vi "play-with-variants_write_to_file.vi"() -> ()   [LabVIEW 2019]
uses:
  <vilib>/Utility/Data Type/Type Definitions/Data Type.ctl
  <vilib>/Utility/Data Type/Type Definitions/Type Definition Info.ctl
  <vilib>/Rock Robotics/SystemInterfaces/NetworkCommunication/NetComm_UsageReport_report.vi
  <vilib>/Rock Robotics/WPI/ThirdParty/JAS_Junk/TrajLib/DiffDriveKinematicsConstraint_New.vi
  <vilib>/Rock Robotics/WPI/ThirdParty/JAS_Junk/TrajLib/TrajectoryConfig_AddConstraint.vi
  <vilib>/Rock Robotics/WPI/ThirdParty/JAS_Junk/TrajLib/CentripetalAccelConstraint_New.vi
  <vilib>/Rock Robotics/WPI/ThirdParty/JAS_Junk/TrajLib/DiffDriveVoltageConstraint_New.vi
  <vilib>/Rock Robotics/WPI/ThirdParty/JAS_Junk/TrajLib/MecaDriveKinematicsConstraint_New.vi
  <vilib>/Rock Robotics/WPI/ThirdParty/JAS_Junk/TrajLib/SwerveDriveKinematicsConstraint_New.vi
  <vilib>/Rock Robotics/WPI/ThirdParty/JAS_Junk/TrajLib/Util_LibraryGlobals.vi
  <vilib>/Rock Robotics/WPI/ThirdParty/JAS_Junk/TrajLib/Trajectory_Library.lvlib
  <vilib>/Utility/Data Type/NI_Data Type.lvlib
  <vilib>/Rock Robotics/WPI/ThirdParty/JAS_Junk/TrajLib/TRAJ_CONSTRAINT_CENTRIPETAL_ACCEL.ctl
  <vilib>/Rock Robotics/WPI/ThirdParty/JAS_Junk/TrajLib/DIFF_DRIVE_KINEMATICS.ctl
  <vilib>/Rock Robotics/WPI/ThirdParty/JAS_Junk/TrajLib/TRAJ_CONSTRAINT_DIIF_DRIVE_KINEMATICS.ctl
  <vilib>/Rock Robotics/WPI/ThirdParty/JAS_Junk/TrajLib/TRANSLATION2D.ctl
  <vilib>/Analysis/Matrix/Datatypes/RealMatrix.ctl
  <vilib>/Analysis/Matrix/NI_Matrix.lvlib
  <vilib>/Rock Robotics/WPI/ThirdParty/JAS_Junk/TrajLib/MECA_DRIVE_KINEMATICS.ctl
  <vilib>/Rock Robotics/WPI/ThirdParty/JAS_Junk/TrajLib/TRAJ_CONSTRAINT_MECA_DRIVE_KINEMATICS.ctl
  <vilib>/Rock Robotics/WPI/ThirdParty/JAS_Junk/TrajLib/SWERVE_DRIVE_KINEMATICS.ctl
  <vilib>/Rock Robotics/WPI/ThirdParty/JAS_Junk/TrajLib/TRAJ_CONSTRAINT_SWERVE_DRIVE_KINEMATICS.ctl
  <vilib>/Rock Robotics/WPI/ThirdParty/JAS_Junk/TrajLib/SIMPLE_MOTOR_FF.ctl
  <vilib>/Rock Robotics/WPI/ThirdParty/JAS_Junk/TrajLib/TRAJ_CONSTRAINT_DIIF_DRIVE_VOLTAGE.ctl
  TrajConfig_XML_V5.ctl
panel:
  out "output cluster":T1 {"CentAccelConstraint"."Max Cent Accel" format="%20.4f"; "DiffDriveKineConstraint"."Max Accel (M/S2)" format="%20.4f"; "DiffDriveKineConstraint"."DIFF_DRIVE_KINEMATICS"."TrackWidth_Meters" format="%20.4f"; "DiffDriveKineConstraint"."Max Speed (M/S)" format="%20.4f"; "MecaKineConstraint"."MECA_DRIVE_KINEMATICS"."PrevCoR"."Y" format="%14.3f"; "MecaKineConstraint"."MECA_DRIVE_KINEMATICS"."PrevCoR"."X" format="%14.3f"; "MecaKineConstraint"."MECA_DRIVE_KINEMATICS"."RearRight"."Y" format="%14.3f"; "MecaKineConstraint"."MECA_DRIVE_KINEMATICS"."RearRight"."X" format="%14.3f"; "MecaKineConstraint"."MECA_DRIVE_KINEMATICS"."RearLeft"."Y" format="%14.3f"; "MecaKineConstraint"."MECA_DRIVE_KINEMATICS"."RearLeft"."X" format="%14.3f"; "MecaKineConstraint"."MECA_DRIVE_KINEMATICS"."FrontRight"."Y" format="%14.3f"; "MecaKineConstraint"."MECA_DRIVE_KINEMATICS"."FrontRight"."X" format="%14.3f"; "MecaKineConstraint"."MECA_DRIVE_KINEMATICS"."FrontLeft"."Y" format="%14.3f"; "MecaKineConstraint"."MECA_DRIVE_KINEMATICS"."FrontLeft"."X" format="%14.3f"; "MecaKineConstraint"."Max Speed (M/S)" format="%20.4f"; "SwerveKineConstraint"."SwerveKinematics"."PrevCoR"."Y" format="%14.3f"; "SwerveKineConstraint"."SwerveKinematics"."PrevCoR"."X" format="%14.3f"; "SwerveKineConstraint"."SwerveKinematics"."Modules"."Y" format="%14.3f"; "SwerveKineConstraint"."SwerveKinematics"."Modules"."X" format="%14.3f"; "SwerveKineConstraint"."Max Speed (M/S)" format="%20.4f"; "DiffVoltConstraint"."SIMPLE_MOTOR_FF"."Ka" format="%13.4f"; "DiffVoltConstraint"."SIMPLE_MOTOR_FF"."Kv" format="%13.4f"; "DiffVoltConstraint"."SIMPLE_MOTOR_FF"."Ks" format="%13.4f"; "DiffVoltConstraint"."DIFF_DRIVE_KINEMATICS"."TrackWidth_Meters" format="%20.4f"; "DiffVoltConstraint"."Max Voltage" format="%20.4f"}
  out "error out":errorcluster
  out "xml string":string
  out "Constraints":variant[](array[variant])
  out "TypeDefInfo":T13[](array[typedef])
  out "TypeDef":bool[](array[boolean])
  out "Name":string[](array[string])
  out "Type":T14[](array[typedef])
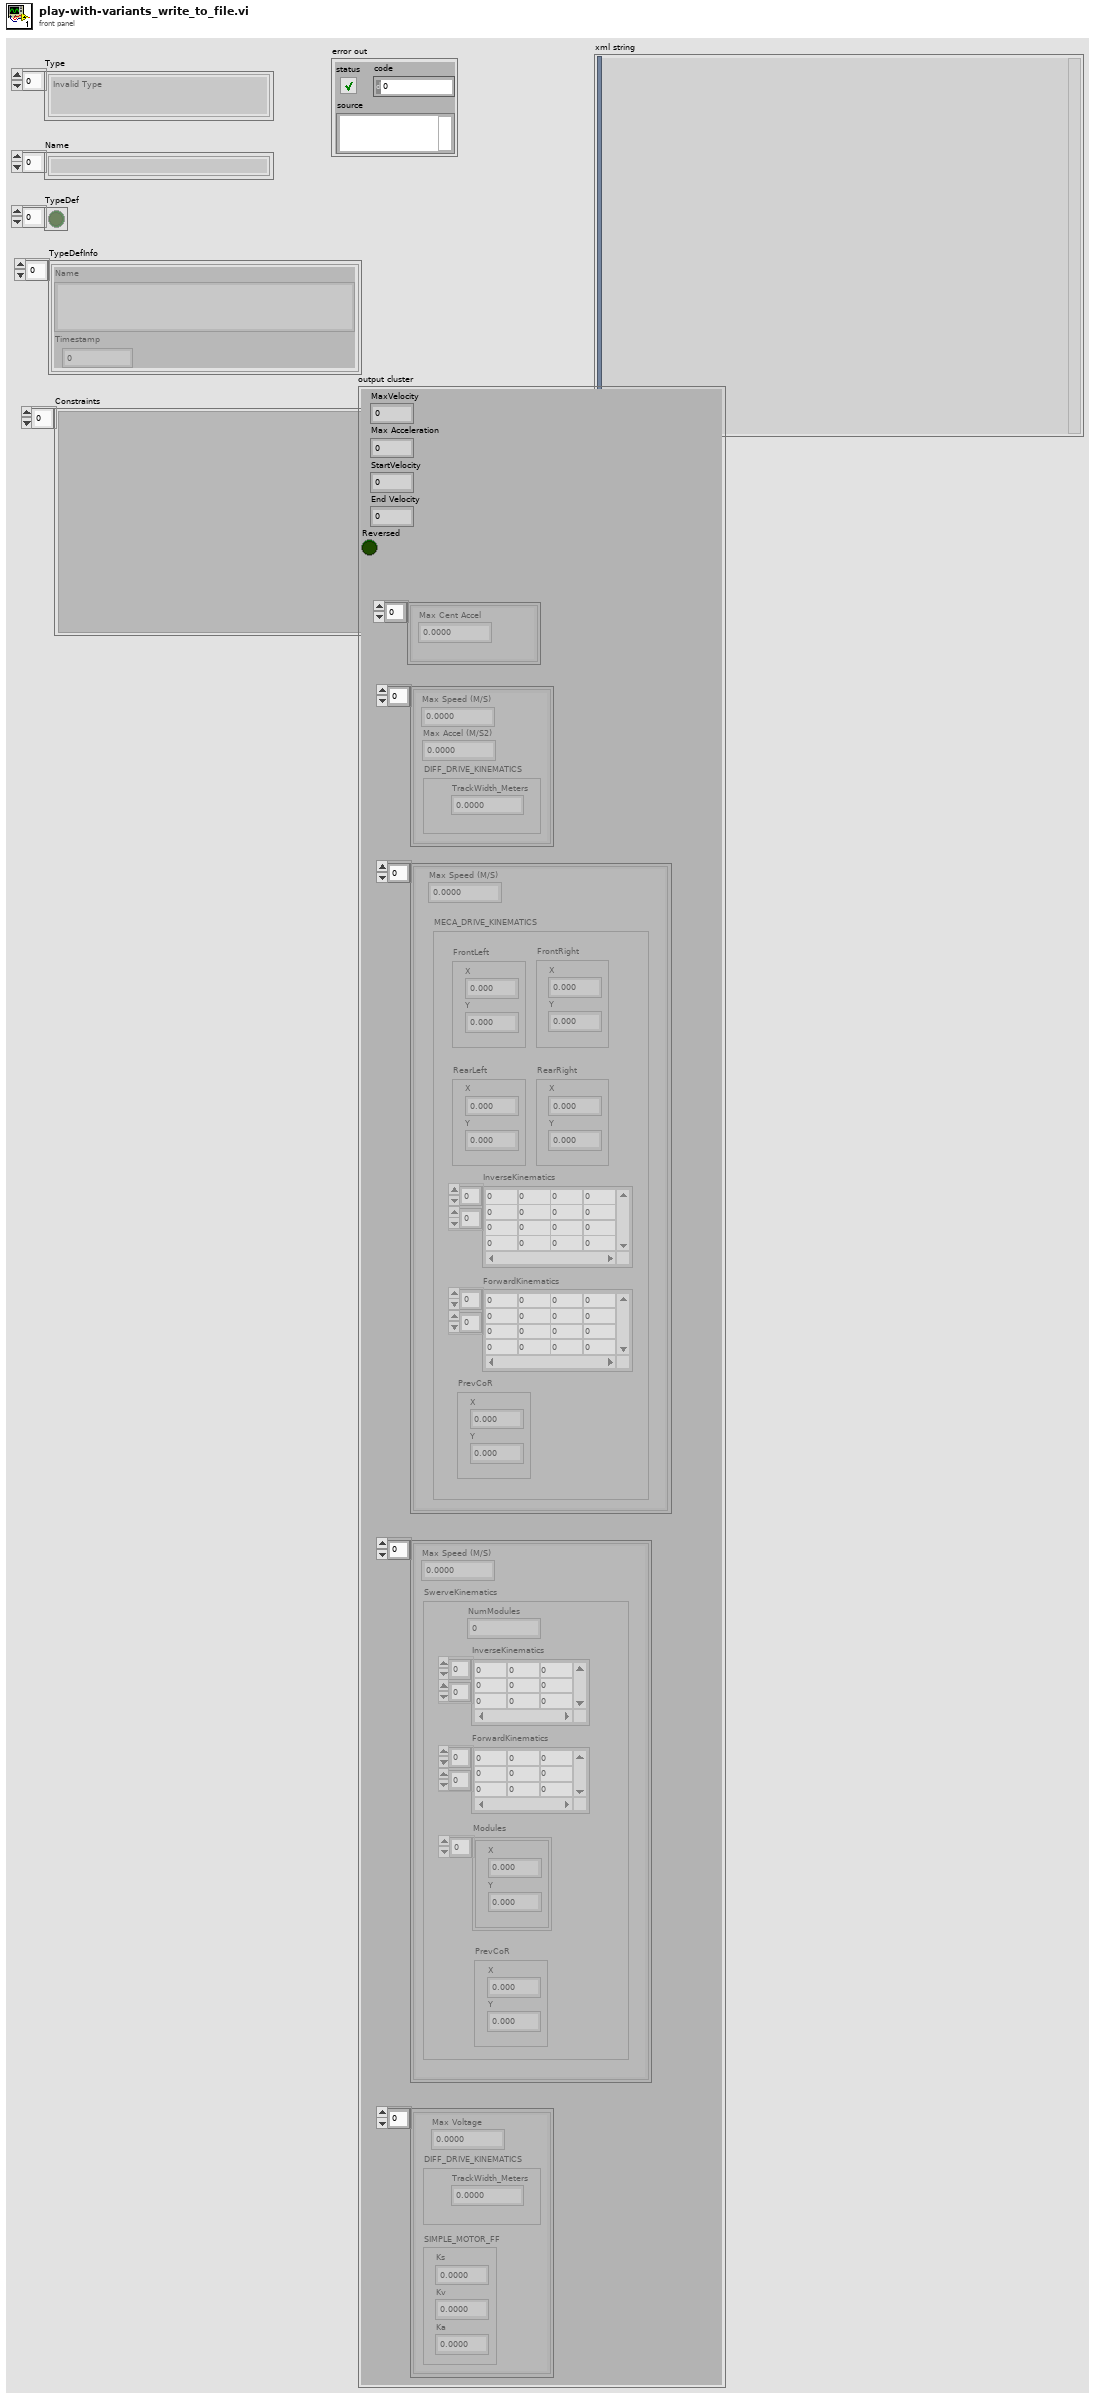
[diagram p1: front panel]
types:
  T1 = typedef "TrajConfig_XML_V5.ctl" = cluster{"MaxVelocity":dbl, "Max Acceleration":dbl, "StartVelocity":dbl, "End Velocity":dbl, "Reversed":bool, "CentAccelConstraint":T2[], "DiffDriveKineConstraint":T3[], "MecaKineConstraint":T5[], "SwerveKineConstraint":T9[], "DiffVoltConstraint":T11[]}
  T2 = typedef "Trajectory_Library.lvlib/TRAJ_CONSTRAINT_CENTRIPETAL_ACCEL.ctl" = cluster{"Max Cent Accel":dbl}
  T3 = typedef "Trajectory_Library.lvlib/TRAJ_CONSTRAINT_DIIF_DRIVE_KINEMATICS.ctl" = cluster{"Max Speed (M/S)":dbl, "DIFF_DRIVE_KINEMATICS":T4, "Max Accel (M/S2)":dbl}
  T4 = typedef "Trajectory_Library.lvlib/DIFF_DRIVE_KINEMATICS.ctl" = cluster{"TrackWidth_Meters":dbl}
  T5 = typedef "Trajectory_Library.lvlib/TRAJ_CONSTRAINT_MECA_DRIVE_KINEMATICS.ctl" = cluster{"Max Speed (M/S)":dbl, "MECA_DRIVE_KINEMATICS":T6}
  T6 = typedef "Trajectory_Library.lvlib/MECA_DRIVE_KINEMATICS.ctl" = cluster{"FrontLeft":T7, "FrontRight":T7, "RearLeft":T7, "RearRight":T7, "InverseKinematics":T8, "ForwardKinematics":T8, "PrevCoR":T7}
  T7 = typedef "Trajectory_Library.lvlib/TRANSLATION2D.ctl" = cluster{"X":dbl, "Y":dbl}
  T8 = typedef "NI_Matrix.lvlib/RealMatrix.ctl" = dbl[][]
  T9 = typedef "Trajectory_Library.lvlib/TRAJ_CONSTRAINT_SWERVE_DRIVE_KINEMATICS.ctl" = cluster{"Max Speed (M/S)":dbl, "SwerveKinematics":T10}
  T10 = typedef "Trajectory_Library.lvlib/SWERVE_DRIVE_KINEMATICS.ctl" = cluster{"NumModules":i32, "InverseKinematics":T8, "ForwardKinematics":T8, "Modules":T7[], "PrevCoR":T7}
  T11 = typedef "Trajectory_Library.lvlib/TRAJ_CONSTRAINT_DIIF_DRIVE_VOLTAGE.ctl" = cluster{"Max Voltage":dbl, "DIFF_DRIVE_KINEMATICS":T4, "SIMPLE_MOTOR_FF":T12}
  T12 = typedef "Trajectory_Library.lvlib/SIMPLE_MOTOR_FF.ctl" = cluster{"Ks":dbl, "Kv":dbl, "Ka":dbl}
  T13 = typedef "NI_Data Type.lvlib/Type Definition Info.ctl" = cluster{"Name":string, "Timestamp":u32}
  T14 = typedef "NI_Data Type.lvlib/Data Type.ctl" = enum8{"Invalid Type", "Void", "I8", "I16", "I32", "I64", "U8", "U16", "U32", "U64", "Single Float", "Double Float", "Extended Float", "Single Complex", "Double Complex", "Extended Complex", "Enum U8", "Enum U16", "Enum U32", "Enum U64", "Single Float With Unit", "Double Float With Unit", "Extended Float With Unit", "Single Complex with Unit", "Double Complex with Unit", "Extended Complex with Unit", "Boolean", "String", "Path", "Picture", "Tag", "Array", "Cluster", "Variant", "LV Variant", "Waveform", "Timestamp", "Digital Waveform", "Digital Data", "ExpressData", "Refnum", "External Data", "VI", "Poly VI", "LabVIEW Class Instance", "Fixed Point", "Set Collection", "Map Collection"}
  T15 = typedef "Trajectory_Library.lvlib/TRAJ_CONFIG.ctl" = cluster{"MaxVelocity":dbl, "Max Acceleration":dbl, "StartVelocity":dbl, "End Velocity":dbl, "Reversed":bool, "Constraints":variant[]}
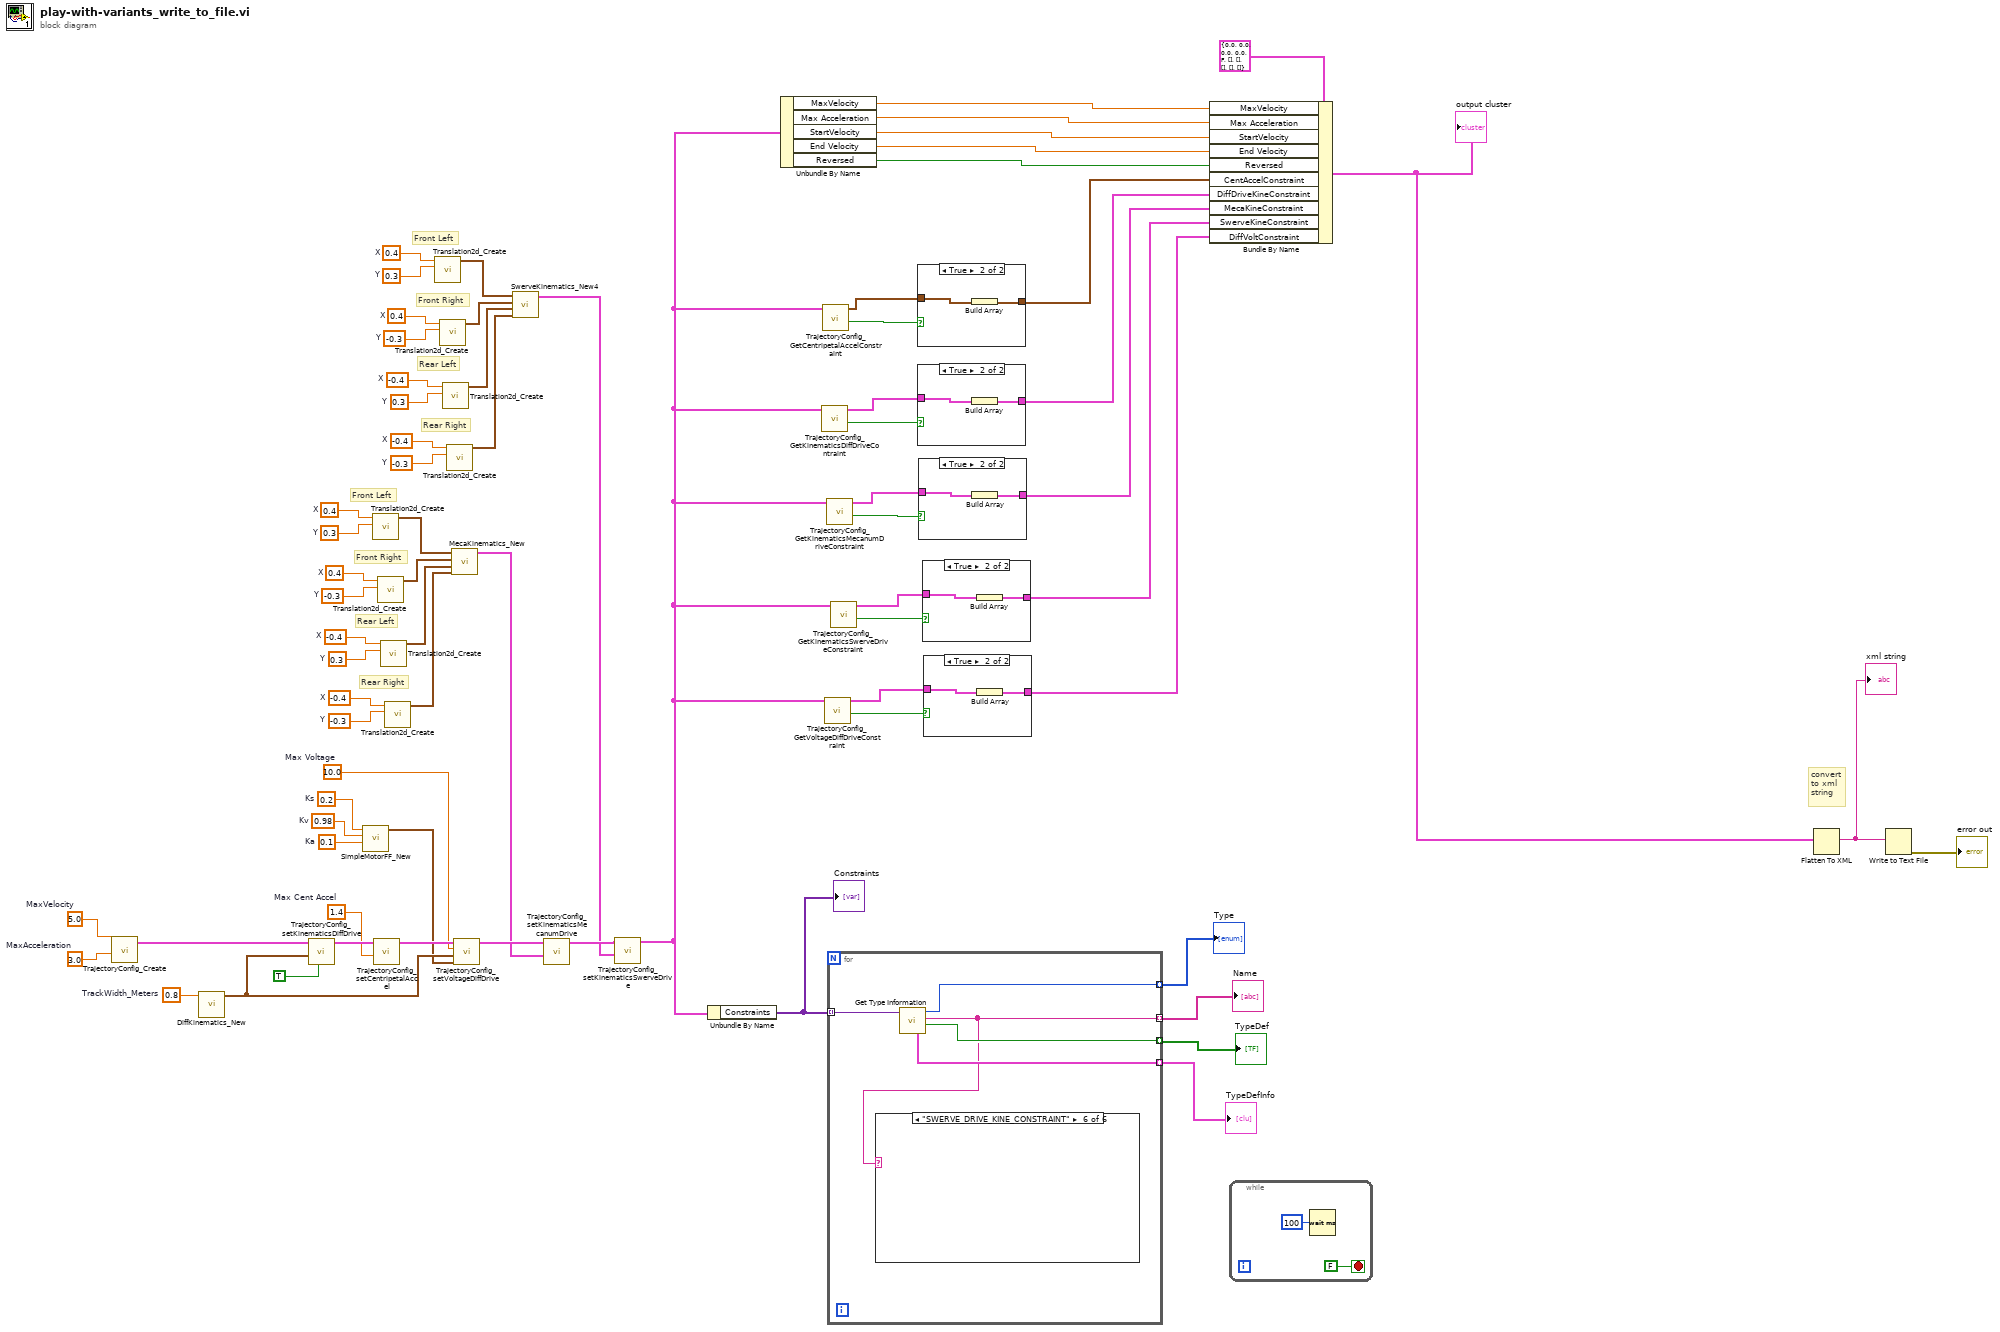
[diagram p0: block diagram]
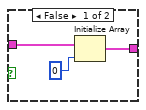
[diagram p2: hidden frame]
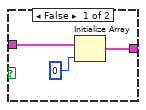
[diagram p3: hidden frame]
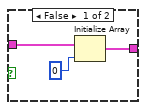
[diagram p4: hidden frame]
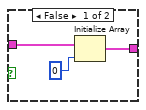
[diagram p5: hidden frame]
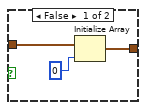
[diagram p6: hidden frame]
diagram:
  w36 = -0.4  # X
  w35 = -0.3  # Y
  w34 = -0.4  # X
  w33 = 0.3  # Y
  w32 = 0.4  # X
  w31 = -0.3  # Y
  w30 = 0.4  # X
  w29 = 0.3  # Y
  w50 = -0.4  # X
  w49 = -0.3  # Y
  w48 = -0.4  # X
  w47 = 0.3  # Y
  w46 = 0.4  # X
  w45 = -0.3  # Y
  w44 = 0.4  # X
  w43 = 0.3  # Y
  w56 = 10.0  # Max Voltage
  w59 = 0.2  # Ks
  w58 = 0.98  # Kv
  w57 = 0.1  # Ka
  w65 = 0.8  # TrackWidth_Meters
  w67 = 5.0  # MaxVelocity
  w68 = 3.0  # MaxAcceleration
  w62 = 1.4  # Max Cent Accel
  # "convert\nto xml\nstring"
  # "Rear Right"
  # "Rear Left"
  # "Front Right"
  # "Front Left"
  # "Rear Right"
  # "Rear Left"
  # "Front Right"
  # "Front Left"
  n1 = call <vilib>:"TrajectoryConfig_Create.vi"("MaxAcceleration"=w68, "MaxVelocity"=w67) -> ("TRAJECTORY_CONFIG"=w66:T15)  [unwired: 9 in]
  n2 = call <vilib>:"DiffKinematics_New.vi"("TrackWidth_Meters"=w65) -> ("DIFF_DRIVE_KINEMATICS"=w60:T4)  [unwired: 10 in]
  n3 = call <vilib>:"TrajectoryConfig_setKinematicsDiffDrive.vi"("Use Accel"=TRUE, "DIFF_DRIVE_KINEMATICS"=w60, "inTRAJECTORY_CONFIG"=w66) -> ("outTRAJECTORY_CONFIG"=w63:T15)  [unwired: 8 in]
  n4 = call <vilib>:"SimpleMotorFF_New.vi"("Ka"=w57, "Kv"=w58, "Ks"=w59) -> ("SIMPLE_MOTOR_FF"=w55:T12)  [unwired: 8 in]
  n5 = call <vilib>:"Translation2d_Create.vi"("Y"=w43, "X"=w44) -> ("TRANSLATION"=w51:T7)  [unwired: 9 in]
  n6 = call <vilib>:"TrajectoryConfig_setCentripetalAccel.vi"("Max Cent Accel"=w62, "inTRAJECTORY_CONFIG"=w63) -> ("outTRAJECTORY_CONFIG"=w61:T15)  [unwired: 9 in]
  n7 = call <vilib>:"Translation2d_Create.vi"("Y"=w45, "X"=w46) -> ("TRANSLATION"=w52:T7)  [unwired: 9 in]
  n8 = call <vilib>:"Translation2d_Create.vi"("Y"=w47, "X"=w48) -> ("TRANSLATION"=w53:T7)  [unwired: 9 in]
  n9 = call <vilib>:"Translation2d_Create.vi"("Y"=w49, "X"=w50) -> ("TRANSLATION"=w54:T7)  [unwired: 9 in]
  n10 = call <vilib>:"Translation2d_Create.vi"("Y"=w29, "X"=w30) -> ("TRANSLATION"=w37:T7)  [unwired: 9 in]
  n11 = call <vilib>:"Translation2d_Create.vi"("Y"=w31, "X"=w32) -> ("TRANSLATION"=w38:T7)  [unwired: 9 in]
  n12 = call <vilib>:"Translation2d_Create.vi"("Y"=w33, "X"=w34) -> ("TRANSLATION"=w39:T7)  [unwired: 9 in]
  n13 = call <vilib>:"Translation2d_Create.vi"("Y"=w35, "X"=w36) -> ("TRANSLATION"=w40:T7)  [unwired: 9 in]
  n14 = call <vilib>:"MecaKinematics_New.vi"("RearRight"=w54, "RearLeft"=w53, "FrontRight"=w52, "FrontLeft"=w51) -> ("MECA_DRIVE_KINEMATICS"=w41:T6)  [unwired: 7 in]
  n15 = call <vilib>:"TrajectoryConfig_setVoltageDiffDrive.vi"("SIMPLE_MOTOR_FF"=w55, "DIFF_DRIVE_KINEMATICS"=w60, "Max Voltage"=w56, "inTRAJECTORY_CONFIG"=w61) -> ("outTRAJECTORY_CONFIG"=w42:T15)  [unwired: 7 in]
  n16 = call <vilib>:"SwerveKinematics_New4.vi"("wheel 3"=w40, "wheel 2"=w39, "wheel 1"=w38, "wheel 0"=w37) -> ("SWERVE_DRIVE_KINEMATICS"=w27:T10)  [unwired: 7 in]
  n17 = call <vilib>:"TrajectoryConfig_setKinematicsMecanumDrive.vi"("MECA_DRIVE_KINEMATICS"=w41, "inTRAJECTORY_CONFIG"=w42) -> ("outTRAJECTORY_CONFIG"=w28:T15)  [unwired: 9 in]
  n18 = call <vilib>:"TrajectoryConfig_setKinematicsSwerveDrive.vi"("SWERVE_DRIVE_KINEMATICS"=w27, "inTRAJECTORY_CONFIG"=w28) -> ("TRAJECTORY_CONFIG"=w23:T15)  [unwired: 9 in]
  n19 = Unbundle By Name(w23) -> ("Constraints"=w26:variant[])
  "Constraints" <- w26
  n20 = Unbundle By Name(w23) -> ("MaxVelocity"=w12:dbl, "Max Acceleration"=w11:dbl, "StartVelocity"=w10:dbl, "End Velocity"=w9:dbl, "Reversed"=w8:bool)
  n21 = call <vilib>:"TrajectoryConfig_GetKinematicsDiffDriveContraint.vi"("inTRAJECTORY_CONFIG"=w23) -> ("Constraint Exists"=w20:bool, "Diff Drive Kinematics Constraint"=w19:T3)  [unwired: 9 in]
  n22 = call <vilib>:"TrajectoryConfig_GetCentripetalAccelConstraint.vi"("inTRAJECTORY_CONFIG"=w23) -> ("Constraint Exists"=w22:bool, "Centripital Accleration Constraint"=w21:T2)  [unwired: 9 in]
  n23 = call <vilib>:"TrajectoryConfig_GetVoltageDiffDriveConstraint.vi"("inTRAJECTORY_CONFIG"=w23) -> ("Constraint Exists"=w14:bool, "Differential Drive Voltage Constraint"=w13:T11)  [unwired: 9 in]
  n24 = call <vilib>:"TrajectoryConfig_GetKinematicsMecanumDriveConstraint.vi"("inTRAJECTORY_CONFIG"=w23) -> ("Constraint Exists"=w18:bool, "Mecanum Drive Kinematics Constraint"=w17:T5)  [unwired: 9 in]
  n25 = for {
    tunnel: [w77] -> w72 mode=indexing
    tunnel: [w74] -> w71 mode=indexing
    tunnel: [w75] -> w70 mode=indexing
    tunnel: [w76] -> w69 mode=indexing
    tunnel: w26 -> [w73] mode=indexing
    n26 = call <vilib>:"Get Type Information.vi"("variant"=w73) -> ("type definition"=w75:bool, "name"=w74:string, "type"=w77:T14, "type definition info"=w76:T13)  [unwired: 6 in, 1 out]
    n27 = case shown="\"SWERVE_DRIVE_KINE_CONSTRAINT\"" w74 {
      frame Default {
      }
      frame "DIFF_DRIVE_KINE_CONSTRAINT" {
      }
      frame "CENTRIPETAL_ACCEL_CONSTRAINT" {
      }
      frame "DIFF_DRIVE_VOLTAGE_CONSTRAINT" {
      }
      frame "MECANUM_DRIVE_KINE_CONSTRAINT" {
      }
      frame "SWERVE_DRIVE_KINE_CONSTRAINT" {
      }
    }
  }
  "Type" <- w72
  "Name" <- w71
  "TypeDef" <- w70
  "TypeDefInfo" <- w69
  n28 = call <vilib>:"TrajectoryConfig_GetKinematicsSwerveDriveConstraint.vi"("inTRAJECTORY_CONFIG"=w23) -> ("Constraint Exists"=w16:bool, "Swerver Drive Kinematics Constraint"=w15:T9)  [unwired: 9 in]
  n29 = case shown="True" w22 {
    tunnel: w21 -> [w80 w82]
    tunnel: [w78 w81] -> w7
    frame False {
      n30 = Initialize Array(w80, 0 ("dimension size")) -> (w78:T2[])
    }
    frame True {
      n31 = Build Array(w82) -> (w81:T2[])
    }
  }
  n32 = case shown="True" w20 {
    tunnel: w19 -> [w85 w87]
    tunnel: [w83 w86] -> w6
    frame False {
      n33 = Initialize Array(w85, 0 ("dimension size")) -> (w83:T3[])
    }
    frame True {
      n34 = Build Array(w87) -> (w86:T3[])
    }
  }
  n35 = case shown="True" w18 {
    tunnel: w17 -> [w90 w92]
    tunnel: [w88 w91] -> w5
    frame False {
      n36 = Initialize Array(w90, 0 ("dimension size")) -> (w88:T5[])
    }
    frame True {
      n37 = Build Array(w92) -> (w91:T5[])
    }
  }
  n38 = case shown="True" w16 {
    tunnel: w15 -> [w95 w97]
    tunnel: [w93 w96] -> w4
    frame False {
      n39 = Initialize Array(w95, 0 ("dimension size")) -> (w93:T9[])
    }
    frame True {
      n40 = Build Array(w97) -> (w96:T9[])
    }
  }
  n41 = case shown="True" w14 {
    tunnel: w13 -> [w100 w102]
    tunnel: [w98 w101] -> w3
    frame False {
      n42 = Initialize Array(w100, 0 ("dimension size")) -> (w98:T11[])
    }
    frame True {
      n43 = Build Array(w102) -> (w101:T11[])
    }
  }
  n44 = Bundle By Name(cluster=T1 {"MaxVelocity"=0.0, "Max Acceleration"=0.0, "StartVelocity"=0.0, "End Velocity"=0.0, "Reversed"=FALSE, "CentAccelConstraint"=[], "DiffDriveKineConstraint"=[], "MecaKineConstraint"=[], "SwerveKineConstraint"=[], "DiffVoltConstraint"=[]} ("TrajConfigXML_V5"), "MaxVelocity"=w12, "Max Acceleration"=w11, "StartVelocity"=w10, "End Velocity"=w9, "Reversed"=w8, "CentAccelConstraint"=w7, "DiffDriveKineConstraint"=w6, "MecaKineConstraint"=w5, "SwerveKineConstraint"=w4, "DiffVoltConstraint"=w3) -> (w2:T1)
  "output cluster" <- w2
  n45 = while {
    stop <- FALSE stop-if-true
    n46 = Wait (ms)(milliseconds to wait=u32 100) -> ()  [unwired: 1 out]
  }
  n47 = Flatten To XML(anything=w2) -> (xml string=w25:string)
  "xml string" <- w25
  n48 = Write to Text File(text=w25) -> (error out=→"error out":errorcluster)  [unwired: 3 in, 2 out]
